vi "Stufen berechnen.vi"(7 "Empfangsdaten":string[](array[string]), 9 "Konzentration":sgl, 11 "Stufen":u16[](array[numeric])) -> (1 "Konzentrationen":sgl[](array[numeric]), 3 "Stufen Tabelle":string[](array[string]))   [LabVIEW 2020, in "Linearisierung v2.lvlib" / "Gasteiler.lvlib" / "AK Komm Gasteiler.lvlib" / "Alter Gasteiler.lvlib"]
uses:
  Alter Gasteiler.lvlib
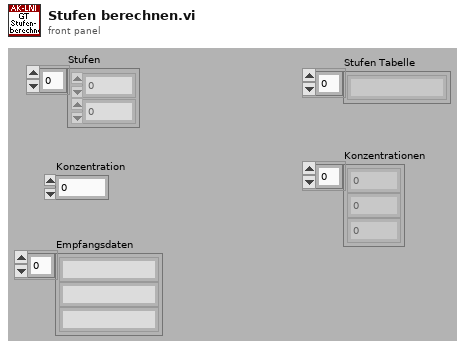
[diagram p1: front panel]
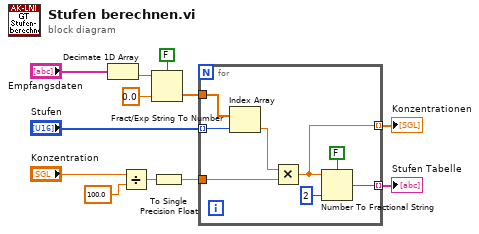
[diagram p0: block diagram]
diagram:
  n1 = Decimate 1D Array("Empfangsdaten") -> (w4:string[])  [unwired: 1 out]
  n2 = Divide(x="Konzentration", y=sgl 100.0) -> (x/y=w10:sgl)
  n3 = Fract/Exp String To Number(use system decimal point (T)=FALSE ("Systemdezimalzeichen verwenden (T)"), string=w4, default (0 dbl)=sgl 0.0 ("y")) -> (number=w1:sgl[])  [unwired: 1 in, 1 out]
  n4 = To Single Precision Float(number=w10) -> (single precision float=w8:sgl)
  n5 = for {
    tunnel: w1 -> [w20]
    tunnel: "Stufen" -> [w19] mode=indexing
    tunnel: w8 -> [w17]
    tunnel: [w14] -> w7 mode=indexing
    tunnel: [w13] -> w6 mode=indexing
    n6 = Index Array(array=w20, index=w19) -> (element=w18:sgl)
    n7 = Multiply(x=w18, y=w17) -> (x*y=w13:sgl)
    n8 = Number To Fractional String(use system decimal point (T)=FALSE ("Systemdezimalzeichen verwenden (T)"), number=w13, precision (6)=i16 2 ("Genauigkeit (6)")) -> (F-format string=w14:string)  [unwired: 1 in]
  }
  "Stufen Tabelle" <- w7
  "Konzentrationen" <- w6
